vi "login credentials FG.vi"(6 "FG action":T1, 8 "error in":errorcluster, 11 "device class":T3={"cDAQ"=TRUE, "cRIO"=TRUE, "Ethernet RIO"=TRUE, "sbRIO"=TRUE, "PXI"=FALSE, "CVS"=FALSE, "Desktop"=FALSE, "FieldPoint"=FALSE, "<No Device Class>"=FALSE}) -> (0 "error out":errorcluster, 3 "login credentials":T2[](array[typedef]))   [LabVIEW 2013, in "tests.lvlib"]
uses:
  tests.lvlib
  classes/Device/device class selection.ctl
  classes/Device/login credentials.ctl
  classes/Device/FG action.ctl
  classes/Device/device login credentials.ctl
  classes/Device/device class.ctl
  <vilib>/regexp/Match Regular Expression.xnode
  classes/Device/Device.lvclass
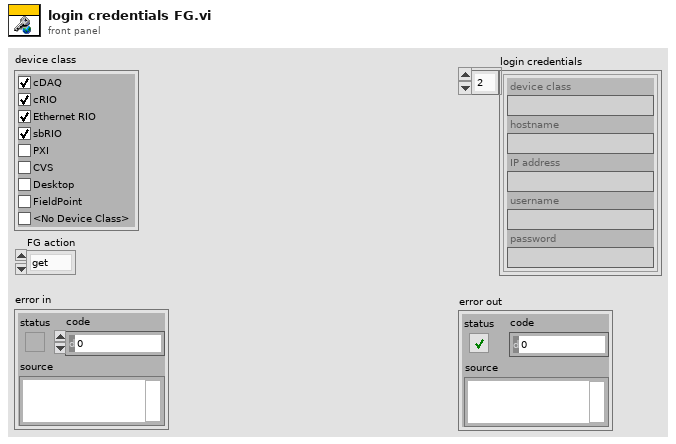
[diagram p1: front panel]
types:
  T1 = typedef "SMI.lvlib/Device.lvclass/FG action.ctl" = enum16{"get", "set"}
  T2 = typedef "SMI.lvlib/Device.lvclass/login credentials.ctl" = cluster{"device class":string, "hostname":string, "IP address":string, "username":string, "password":string}
  T3 = typedef "SMI.lvlib/Device.lvclass/device class selection.ctl" = cluster{"cDAQ":bool, "cRIO":bool, "Ethernet RIO":bool, "sbRIO":bool, "PXI":bool, "CVS":bool, "Desktop":bool, "FieldPoint":bool, "<No Device Class>":bool}
  T4 = typedef "SMI.lvlib/Device.lvclass/device login credentials.ctl" = cluster{"device class":T5, "hostname regular expression":string, "username":string, "password":string}
  T5 = typedef "SMI.lvlib/Device.lvclass/device class.ctl" = enum16{"cDAQ", "cRIO", "Ethernet RIO", "sbRIO", "PXI", "CVS", "Desktop", "FieldPoint", "<No Device Class>", "<Detect All>"}
  T6 = typedef "SMI.lvlib/Device.lvclass/network device information.ctl" = cluster{"hostname":string, "IP address":string, "MAC address":string, "vendor name":string, "product name":string, "product ID":u16, "serial number":string, "device class":string}
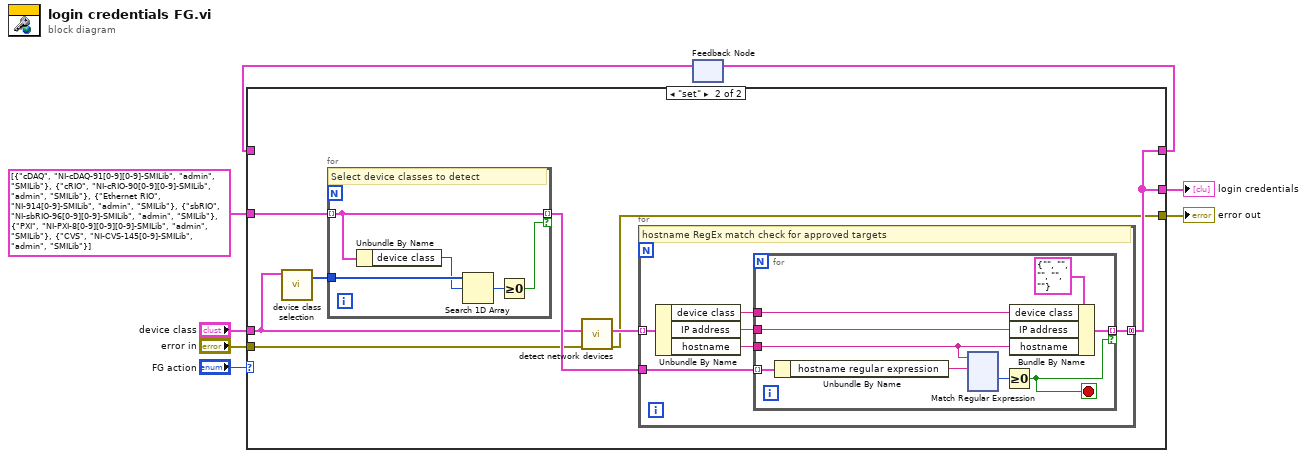
[diagram p0: block diagram]
diagram:
  n1 = feedback #1() -> (w6:T2[])  [unwired: 1 in]
  n2 = case shown="\"set\"" "FG action" {
    tunnel: "device class" -> [_ w14]
    tunnel: [w10 w15] -> w7
    tunnel: w6 -> [w10 _]
    tunnel: [w10 w15] -> w5
    tunnel: [w9 w13] -> w3
    tunnel: "error in" -> [w9 w11]
    tunnel: T4[] [{"device class"=enum."cDAQ", "hostname regular expression"="NI-cDAQ-91[0-9][0-9]-SMILib", "username"="admin", "password"="SMILib"}, {"device class"=enum."cRIO", "hostname regular expression"="NI-cRIO-90[0-9][0-9]-SMILib", "username"="admin", "password"="SMILib"}, {"device class"=enum."Ethernet RIO", "hostname regular expression"="NI-914[0-9]-SMILib", "username"="admin", "password"="SMILib"}, {"device class"=enum."sbRIO", "hostname regular expression"="NI-sbRIO-96[0-9][0-9]-SMILib", "username"="admin", "password"="SMILib"}, {"device class"=enum."PXI", "hostname regular expression"="NI-PXI-8[0-9][0-9][0-9]-SMILib", "username"="admin", "password"="SMILib"}, {"device class"=enum."CVS", "hostname regular expression"="NI-CVS-145[0-9]-SMILib", "username"="admin", "password"="SMILib"}] -> [_ w12]
    frame "get", Default {
    }
    frame "set" {
      n3 = call "device class selection.vi"("device classes"=w14) -> ("device class"=w18:T5[])  [unwired: 6 in]
      n4 = for {
        tunnel: [w148] -> w16 mode=indexing if=w150
        tunnel: w18 -> [w152]
        tunnel: w12 -> [w148] mode=indexing
        # "Select device classes to detect"
        n5 = Unbundle By Name(w148) -> ("device class"=w149:T5)
        n6 = Search 1D Array(1D array=w152, element=w149) -> (index of element=w151:i32)  [unwired: 1 in]
        n7 = Greater Or Equal To 0?(x=w151) -> (x >= 0?=w150:bool)
      }
      n8 = call "detect network devices.vi"("error in"=w11, "device class"=w14) -> ("error out"=w13:errorcluster, "devices"=w17:T6[])  [unwired: 7 in, 1 out]
      n9 = for {
        tunnel: w17 -> [w24] mode=indexing
        tunnel: w16 -> [w23]
        tunnel: [w21] -> w15 mode=concatenating
        # "hostname RegEx match check for approved targets"
        n10 = Unbundle By Name(w24) -> ("device class"=w19:string, "IP address"=w20:string, "hostname"=w22:string)
        n11 = for {
          tunnel: w23 -> [w32] mode=indexing
          tunnel: w22 -> [w27]
          tunnel: [w31] -> w21 mode=indexing if=w25
          tunnel: w20 -> [w29]
          tunnel: w19 -> [w28]
          stop <- w25 stop-if-true
          n12 = Unbundle By Name(w32) -> ("hostname regular expression"=w33:string)
          n13 = xnode "Match Regular Expression"("input string"=w27, "regular expression"=w33) -> ("offset past match"=w30:i32)  [unwired: 4 in, 4 out]
          n14 = Greater Or Equal To 0?(x=w30) -> (x >= 0?=w25:bool)
          n15 = Bundle By Name(cluster=T2 {"device class"="", "hostname"="", "IP address"="", "username"="", "password"=""} ("login credentials"), "device class"=w28, "IP address"=w29, "hostname"=w27) -> (w31:T2)
        }
      }
    }
  }
  "login credentials" <- w5
  "error out" <- w3
  n16 = feedback-in #1(w7) -> ()
